vi "Start.vi"(8 "error in (no error)":errorcluster, 11 "reference in":refnum<class "Test_Flux_Capacitor.lvclass">) -> (0 "error out":errorcluster, 3 "reference in":refnum<class "Test_Flux_Capacitor.lvclass">)   [LabVIEW 2022 SP3, in "Test_Flux_Capacitor.lvlib" / "Test_Flux_Capacitor.lvclass"]
uses:
  Test_Flux_Capacitor.lvclass
  Components/SwitchBase.lvlibp/SwitchBase.lvclass
  Components/PSU_Base.lvlibp/PSU_Base.lvclass
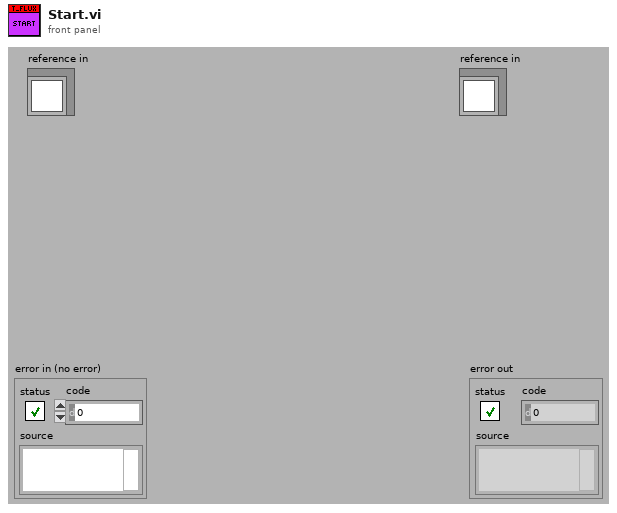
[diagram p1: front panel]
types:
  T1 = typedef "Test_Flux_Capacitor.lvlib/Test_Flux_Capacitor.lvclass/ObjectAttributes.ctl" = cluster{"Config":T2, "DMM":refnum<class "DMM_Keysight_34980A.lvclass">, "LCR":refnum<class "LCR_BK891.lvclass">, "PSU":refnum<class "PSU_Base.lvclass">, "Switch_Manager":refnum<class "SwitchBase.lvclass">, "FRAM":string, "Flux_Capacitor":refnum<class "Flux_Capacitor.lvclass">, "Frequency_Counter":refnum<class "Frequency_Counter_Base.lvclass">, "JTAG":refnum<class "JTAG_Base.lvclass">}
  T2 = typedef "Test_Flux_Capacitor.lvlib/Test_Flux_Capacitor.lvclass/Config.ctl" = cluster{"default":string}
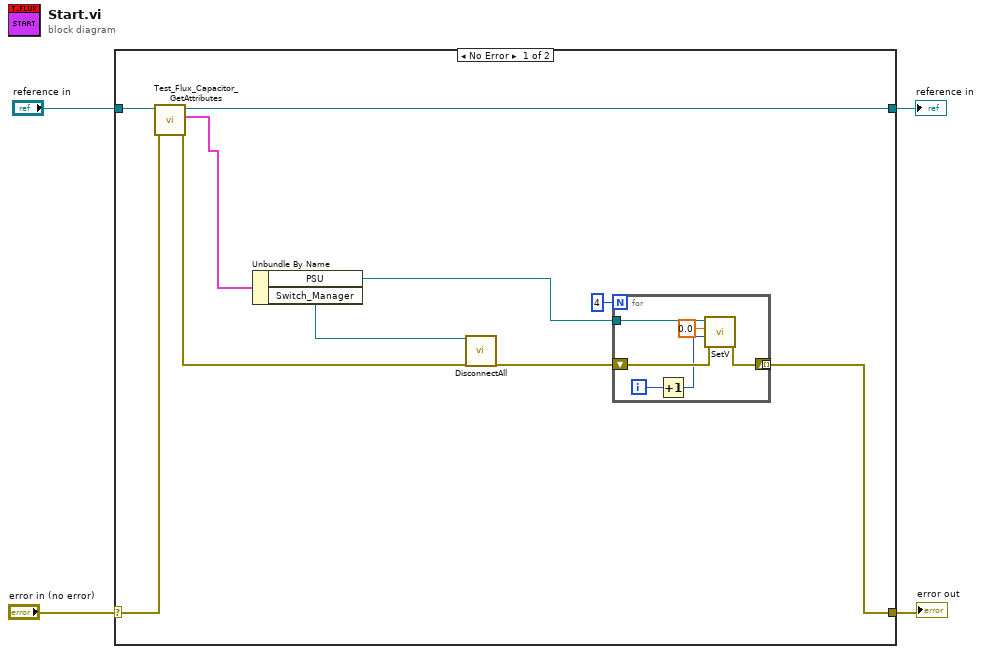
[diagram p0: block diagram]
diagram:
  n1 = case shown="No Error" "error in (no error)" {
    selector: "error in (no error)" -> [w14 w22]
    tunnel: [w5 w22] -> w3
    tunnel: [w12 w21] -> w1
    tunnel: "reference in" -> [w13 w21]
    frame No Error {
      n2 = call "Test_Flux_Capacitor_GetAttributes.vi"("error in (no error)"=w14, "reference in"=w13) -> ("error out"=w6:errorcluster, "Data"=w7:T1, "reference out"=w12:refnum<class "Test_Flux_Capacitor.lvclass">)  [unwired: 6 in, 1 out]
      n3 = Unbundle By Name(w7) -> ("PSU"=w10:refnum<class "PSU_Base.lvclass">, "Switch_Manager"=w11:refnum<class "SwitchBase.lvclass">)
      n4 = call-dynamic "DisconnectAll.vi"("reference in"=w11, "error in (no error)"=w6) -> ("error out"=w8:errorcluster)  [unwired: 16 in, 1 out]
      n5 = for {
        N: 4 -> [_]
        tunnel: w10 -> [w20]
        shift-right: [w15] -> w5
        shift-left: w8 -> [w19]
        tunnel: [w15] -> _ mode=indexing
        i -> [w18]
        n6 = Increment(x=w18) -> (x+1=w17:i32)
        n7 = call-dynamic "SetV.vi"("error in (no error)"=w19, "Chan"=w17, "V"=0.0, "reference in"=w20) -> ("error out"=w15:errorcluster)  [unwired: 6 in, 1 out]
      }
    }
    frame Error {
    }
  }
  "error out" <- w3
  "reference in" <- w1
